vi "NT Read and Format as String.vi"(11 "Name":string="Boolean") -> (3 "Formatted String":string)   [LabVIEW 2017]
doc: "Read the named network table entry and return the data formatted as a string."
panel:
  in  "error in":errorcluster
  out "error out":errorcluster
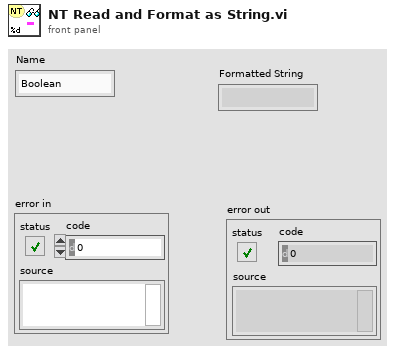
[diagram p1: front panel]
types:
  T1 = typedef "Field Data.ctl" = cluster{"Dbl":dbl, "String":string, "Type":T2, "Boolean":bool, "Sequence #":T3, "Flags":u8}
  T2 = typedef "Field Type.ctl" = enum8{"Invalid", "Bool", "Numeric", "String", "Raw", "Boolean Array", "Numeric Array", "String Array", "RPC"}
  T3 = typedef "Sequence.ctl" = u16
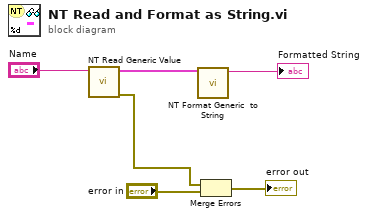
[diagram p0: block diagram]
diagram:
  n1 = call <vilib>:"NT Read Generic Value.vi"("Name"="Name") -> ("error out"=w2:errorcluster, "Field Value"=w6:T1)  [unwired: 9 in]
  n2 = call <vilib>:"NT Format Generic  to String.vi"("Field Value"=w6) -> ("String"=→"Formatted String":string)  [unwired: 10 in]
  n3 = Merge Errors(w2, "error in") -> (→"error out":errorcluster)
